vi "NI_FPGA_PPG.get pdc standby time.vi"(0 "i ref in":refnum<vi>, 5 "error in (no error)":errorcluster) -> (14 "i ref out":refnum<vi>, 16 "pdc_standby":i32, 19 "error out":errorcluster)   [LabVIEW 2014, in "NI_FPGA_PPG.lvlib"]
doc: "Gets PDC standby time specified in the database.\n\nLicense Agreement for this software:\n\nCopyright (C) 2009\nFalk Ziegler\nInstitut für Physik\nErnst-Moritz-Arndt Universität\nFelix-Hausdorff-Str. 6\n17487 Greifswald\n\nContact: Falk Ziegler, ziegler@physik.uni-greifswald.de\n\nThis program is free software: you can redistribute it and/or modify it under the terms of the GNU General Public License as published by the Free Software Foundation, either version 3 of the License, or (at your option) any later version.\n\nThis program is distributed in the hope that it will be useful, but WITHOUT ANY WARRANTY; without even the implied warranty of MERCHANTABILITY or FITNESS FOR A PARTICULAR PURPOSE. See the GNU General Public License for more details.\n\nYou should have received a copy of the GNU General Public License along with this program. If not, see <http://www.gnu.org/licenses/>.\n\nFor all questions and ideas contact: ziegler@physik.uni-greifswald.de or d.beck@gsi.de\nLast update: 01-Sep-2009"
uses:
  NI_FPGA_PPG.lvlib
  CS_Core/BaseProcess/BaseProcess.lvlib
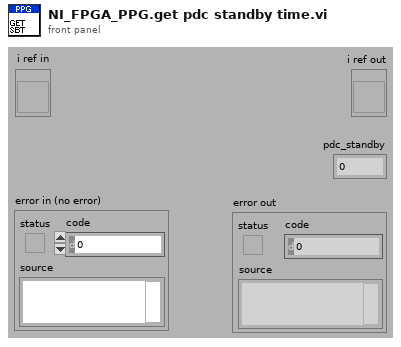
[diagram p1: front panel]
types:
  T1 = typedef "BaseProcess.lvlib/BaseProcess.i attribute.ctl" = cluster{"EventStatus":string, "EventError":i32, "PresetEvtWatchD":i32, "PresetPdcWatchD":i32, "EventTimeout":i32, "PeriodicInterval":i32, "Interface":string[], "Address":string[], "Special":string[], "PeriodicError":i32, "PeriodicStatus":string, "SuperProc":string, "Descriptors":T2[], "CaseRef":refnum<vi>, "PdcRef":refnum<vi>, "Thread Ref":refnum<vi>, "eventErrorID":i32, "eventStatusID":i32, "periodicErrorID":i32, "periodicStatusID":i32, "pdcCtrID":i32}
  T2 = typedef "BaseProcess.lvlib/BaseProcess.descriptor definition.ctl" = cluster{"selector":string, "descriptor":T3}
  T3 = typedef "BaseProcess.lvlib/BaseProcess.descriptor string definition.ctl" = string
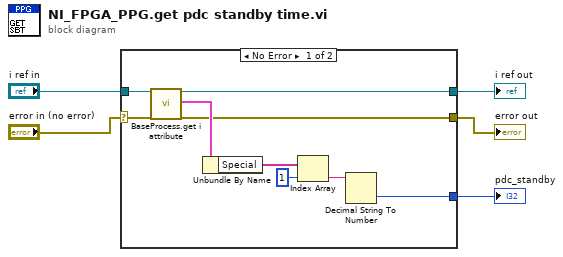
[diagram p0: block diagram]
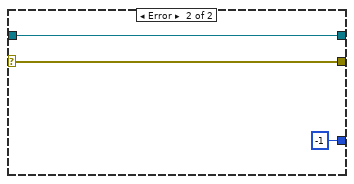
[diagram p2: hidden frame]
diagram:
  n1 = case shown="No Error" "error in (no error)" {
    selector: "error in (no error)" -> [w13 w16]
    tunnel: "i ref in" -> [w14 w17]
    tunnel: [w8 w17] -> w3
    tunnel: [w9 w16] -> w2
    tunnel: [w6 -1] -> w1
    frame No Error {
      n2 = call "BaseProcess.get i attribute.vi"("i ref in"=w14, "error in (no error)"=w13) -> ("i ref out"=w8:refnum<vi>, "i attribute"=w12:T1, "error out"=w9:errorcluster)  [unwired: 15 in]
      n3 = Unbundle By Name(w12) -> ("Special"=w11:string[])
      n4 = Index Array(array=w11, index=1 ("Index")) -> (element=w7:string)
      n5 = Decimal String To Number(string=w7) -> (number=w6:i32)  [unwired: 2 in, 1 out]
    }
    frame Error {
    }
  }
  "error out" <- w2
  "i ref out" <- w3
  "pdc_standby" <- w1
